vi "Queue EXIT state.vi"(1 "Exit Parameters":variant) -> (0 "Exit State Q":T1[](array[typedef]))   [LabVIEW 2013, in "State Machine Lib.lvlib"]
doc: "Builds an exit state with parameters"
uses:
  State Machine Lib.lvlib
  STATE cluster.ctl
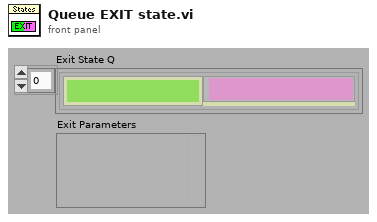
[diagram p1: front panel]
types:
  T1 = typedef "State Machine Lib.lvlib/STATE cluster.ctl" = cluster{"State":string, "Parameters":variant}
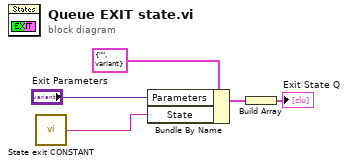
[diagram p0: block diagram]
diagram:
  n1 = call "State exit CONSTANT.vi"() -> ("Exit state"=w1:string)
  n2 = Bundle By Name(cluster=T1 {"State"="", "Parameters"=variant} ("STATE"), "Parameters"="Exit Parameters", "State"=w1) -> (w4:T1)
  n3 = Build Array(w4) -> (→"Exit State Q":T1[])
